vi "LabVIEW Servo Control Proiect.vi"() -> ()   [LabVIEW 2021]
uses:
  <vilib>/MakerHub/LINX/Public/Utilities/Open Serial.vi
  <vilib>/MakerHub/LINX/Public/Sensors/Motion/Servo/Servo Open One Channel.vi
  <vilib>/MakerHub/LINX/Public/Sensors/Motion/Servo/Servo Set Pulse Width One Channel.vi
  <vilib>/MakerHub/LINX/Public/Sensors/Motion/Servo/Servo Close One Channel.vi
  <vilib>/MakerHub/LINX/LMH-LINX.lvlib
  <vilib>/MakerHub/LINX/Public/Sensors/Motion/Servo/Servo.lvlib
panel:
  out "Angle (°)":dbl
  in  "PWM (µS)":u16(slide)=450 min=450 max=2450 step=50 scale=450.0..2450.0
  out "Device Name":string
  in  "Stop":bool
  # "Servo Controls"
  # "General Controls"
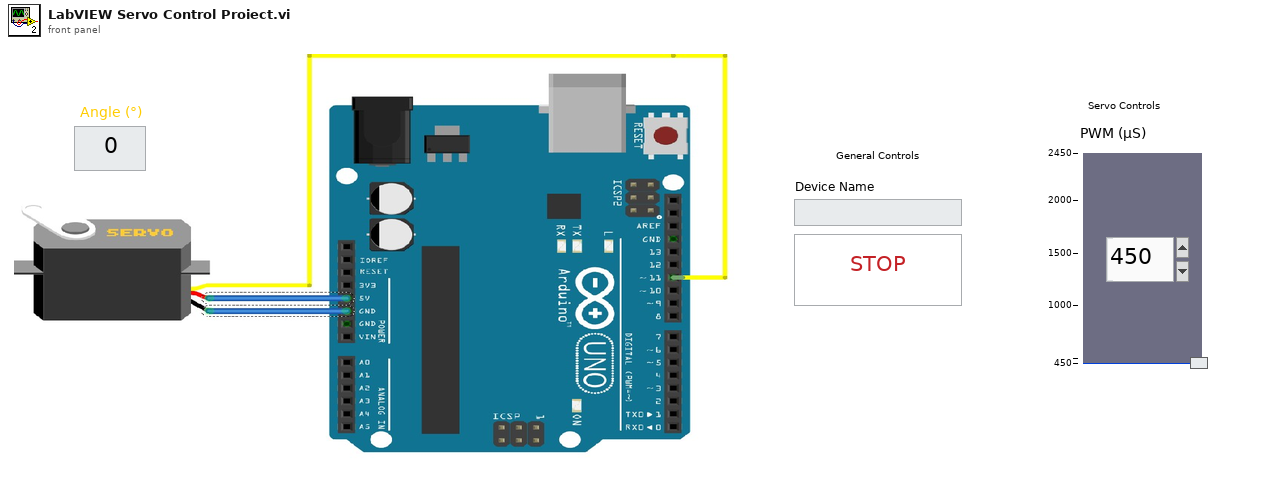
[diagram p1: front panel]
types:
  T1 = typedef "LMH-LINX.lvlib/LINX Ref.ctl" = cluster{"IO":T2, "Interface":T3, "LINX Device Config":T4}
  T2 = typedef "LMH-LINX.lvlib/Platform.ctl" = enum16{"Remote", "Local"}
  T3 = typedef "LMH-LINX.lvlib/Interface.ctl" = enum16{"Serial", "TCP"}
  T4 = typedef "LMH-LINX.lvlib/Device.lvlib/LINX Device Config.ctl" = cluster{"Interface":T3, "COM Port":refnum<visa-resource-name>, "TCP Configuration":T5, "Device Family":u8, "Device ID":u8, "Device Name":string, "TCP Ref":refnum<k5>, "Channels":T6}
  T5 = typedef "LMH-LINX.lvlib/Device.lvlib/TCP Config.ctl" = cluster{"IP Address":string, "Port":u16}
  T6 = typedef "LMH-LINX.lvlib/Channels.ctl" = cluster{"DI":u8[], "DO":u8[], "AI":u8[], "AO":u8[], "PWM":u8[], "QE":u8[], "UART":u8[], "I2C 2":u8[], "SPI":u8[], "CAN":u8[], "Servo":u8[], "AI Ref (V)":dbl, "AI Resolution (Bits)":u8, "AO Ref (V)":dbl, "AO Resolution (Bits)":u8}
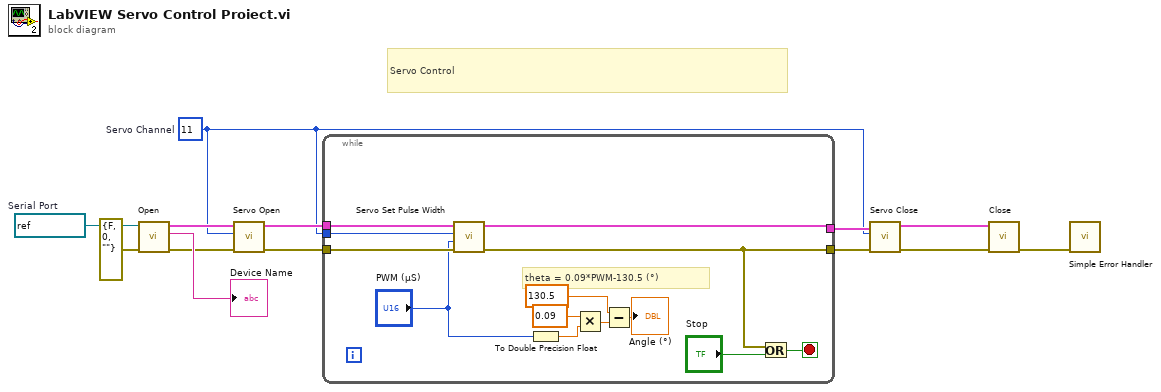
[diagram p0: block diagram]
diagram:
  w1 = u8 11  # Servo Channel
  w13 = refnum<visa-resource-name> "COM3"  # Serial Port
  # "Servo Control"
  n1 = call-poly <vilib>:"Open.vi"("Error In"=errorcluster {"status"=FALSE, "code"=0, "source"=""}, "Serial Port"=w13) -> ("Error Out"=w6:errorcluster, "Device Name"=→"Device Name":string, "LINX Resource"=w7:T1)  [unwired: 7 in]
  n2 = call-poly <vilib>:"Servo Open.vi"("Error In"=w6, "Servo Channel"=w1, "LINX Resource"=w7) -> ("Error Out"=w4:errorcluster, "LINX Resource"=w5:T1)  [unwired: 7 in]
  n3 = while {
    tunnel: [w15] -> w9
    tunnel: [w16] -> w8
    tunnel: w5 -> [w24]
    tunnel: w4 -> [w23]
    tunnel: w1 -> [w14]
    stop <- w25 stop-if-true
    # "theta = 0.09*PWM-130.5 (°)"
    n4 = call-poly <vilib>:"Servo Set Pulse Width.vi"("Error In"=w23, "Pulse Width (uS)"="PWM (µS)", "Servo Channel"=w14, "LINX Resource"=w24) -> ("Error Out"=w16:errorcluster, "LINX Resource"=w15:T1)  [unwired: 6 in]
    n5 = To Double Precision Float(number="PWM (µS)") -> (double precision float=w20:dbl)
    n6 = Multiply(x=0.09, y=w20) -> (x*y=w18:dbl)
    n7 = Subtract(x=130.5, y=w18) -> (x-y=→"Angle (°)":dbl)
    n8 = Or(x=w16, y="Stop") -> (x .or. y?=w25:bool)
  }
  n9 = call-poly <vilib>:"Servo Close.vi"("Error In"=w8, "Servo Channel"=w1, "LINX Resource"=w9) -> ("Error Out"=w3:errorcluster, "LINX Resource"=w2:T1)  [unwired: 7 in]
  n10 = call <vilib>:"Close.vi"("Error In"=w3, "LINX Resource"=w2) -> ("Error Out"=w10:errorcluster)  [unwired: 9 in]
  n11 = call <vilib>:"Simple Error Handler.vi"("error in (no error)"=w10) -> ()  [unwired: 4 in, 5 out]
